vi "File_Header_Ext_VI_Example.vi"() -> (0 "Array":string[][](array[string]))   [LabVIEW 2021]
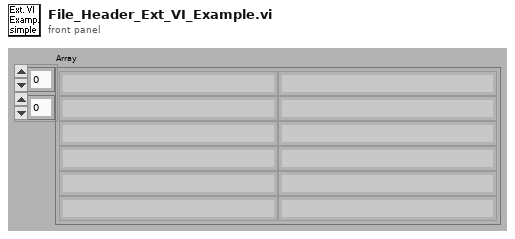
[diagram p1: front panel]
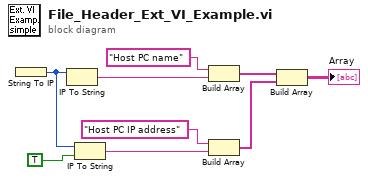
[diagram p0: block diagram]
diagram:
  n1 = String To IP() -> (0:w3:u32)  [unwired: 1 in]
  n2 = IP To String(2:w3) -> (0:w2:string)  [unwired: 1 in]
  n3 = IP To String(1:TRUE ("dot notation? (F)"), 2:w3) -> (0:w1:string)
  n4 = Build Array("Host PC name", w2) -> (w7:string[])
  n5 = Build Array("Host PC IP address", w1) -> (w6:string[])
  n6 = Build Array(w7, w6) -> (→"Array":string[][])
